vi "vna read settings.vi"() -> ()   [LabVIEW 2013]
uses:
  <vilib>/Utility/config.llb/Read Key (Boolean).vi
  <vilib>/Utility/config.llb/Read Key (String).vi
  <vilib>/Utility/config.llb/Read Key (I32).vi
  <vilib>/Utility/config.llb/Read Key (Double).vi
  <vilib>/Utility/config.llb/NI_LVConfig.lvlib
panel:
  out "vna settings":T1
  out "error out":errorcluster
  in  "error in (no error)":errorcluster
  in  "vna settings file":path
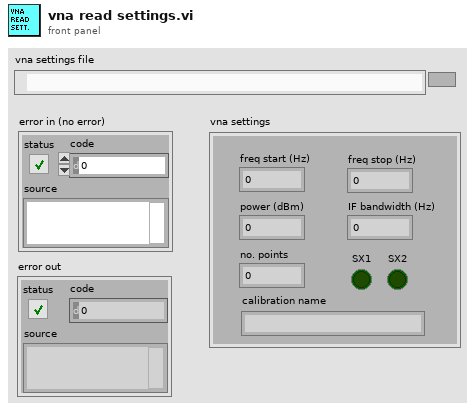
[diagram p1: front panel]
types:
  T1 = cluster{"freq start (Hz)":dbl, "freq stop (Hz)":dbl, "power (dBm)":i32, "IF bandwidth (Hz)":dbl, "no. points":i32, "calibration name":string, "SX1":bool, "SX2":bool}
  T2 = typedef "NI_LVConfig.lvlib/Config Data RefNum.ctl" = refnum<k1>
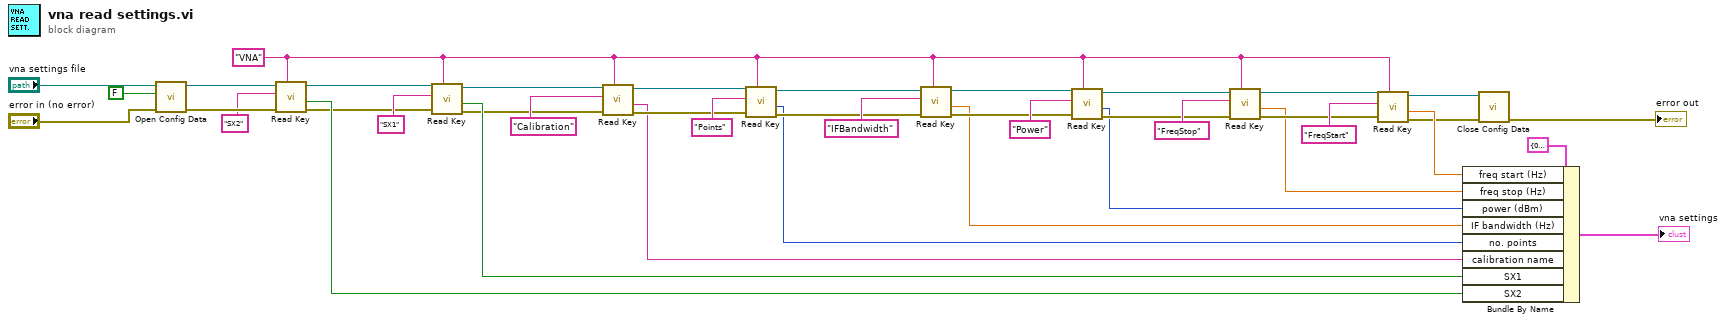
[diagram p0: block diagram]
diagram:
  w1 = "VNA"
  n1 = call <vilib>:"Open Config Data.vi"("error in (no error)"="error in (no error)", "create file if necessary (T)"=FALSE, "configuration file path"="vna settings file") -> ("error out"=w37:errorcluster, "refnum"=w36:T2)  [unwired: 6 in, 1 out]
  n2 = call-poly <vilib>:"Read Key.vi"("section"=w1, "error in (no error)"=w37, "key"="SX2", "refnum"=w36) -> ("error out"=w31:errorcluster, "value"=w34:bool, "refnum out"=w32:T2)  [unwired: 4 in, 1 out]
  n3 = call-poly <vilib>:"Read Key.vi"("section"=w1, "error in (no error)"=w31, "key"="SX1", "refnum"=w32) -> ("error out"=w20:errorcluster, "value"=w30:bool, "refnum out"=w21:T2)  [unwired: 4 in, 1 out]
  n4 = call-poly <vilib>:"Read Key.vi"("section"=w1, "error in (no error)"=w20, "key"="Calibration", "refnum"=w21) -> ("error out"=w26:errorcluster, "value"=w17:string, "refnum out"=w27:T2)  [unwired: 4 in, 1 out]
  n5 = call-poly <vilib>:"Read Key.vi"("section"=w1, "error in (no error)"=w26, "key"="Points", "refnum"=w27) -> ("error out"=w18:errorcluster, "value"=w16:i32, "refnum out"=w19:T2)  [unwired: 4 in, 1 out]
  n6 = call-poly <vilib>:"Read Key.vi"("section"=w1, "error in (no error)"=w18, "key"="IFBandwidth", "refnum"=w19) -> ("error out"=w22:errorcluster, "value"=w15:dbl, "refnum out"=w23:T2)  [unwired: 4 in, 1 out]
  n7 = call-poly <vilib>:"Read Key.vi"("section"=w1, "error in (no error)"=w22, "key"="Power", "refnum"=w23) -> ("error out"=w10:errorcluster, "value"=w8:i32, "refnum out"=w12:T2)  [unwired: 4 in, 1 out]
  n8 = call-poly <vilib>:"Read Key.vi"("section"=w1, "error in (no error)"=w10, "key"="FreqStop", "refnum"=w12) -> ("error out"=w9:errorcluster, "value"=w7:dbl, "refnum out"=w11:T2)  [unwired: 4 in, 1 out]
  n9 = call-poly <vilib>:"Read Key.vi"("section"=w1, "error in (no error)"=w9, "key"="FreqStart", "refnum"=w11) -> ("error out"=w3:errorcluster, "value"=w6:dbl, "refnum out"=w4:T2)  [unwired: 4 in, 1 out]
  n10 = Bundle By Name(cluster=T1 {"freq start (Hz)"=0.0, "freq stop (Hz)"=0.0, "power (dBm)"=0, "IF bandwidth (Hz)"=0.0, "no. points"=0, "calibration name"="", "SX1"=FALSE, "SX2"=FALSE} ("vna settings"), "freq start (Hz)"=w6, "freq stop (Hz)"=w7, "power (dBm)"=w8, "IF bandwidth (Hz)"=w15, "no. points"=w16, "calibration name"=w17, "SX1"=w30, "SX2"=w34) -> (→"vna settings":T1)
  n11 = call <vilib>:"Close Config Data.vi"("error in (no error)"=w3, "refnum"=w4) -> ("error out"=→"error out":errorcluster)  [unwired: 8 in, 1 out]
